vi "Build SMU Waveform.vi"(0 "Measure Load Current":T1, 5 "Record Length":i32, 7 "Source Delay":dbl) -> (4 "SMU Waveform":cluster{dbl[], dbl[]})   [LabVIEW 2020, in "LDO Load Transient.lvlib"]
uses:
  LDO Load Transient.lvlib
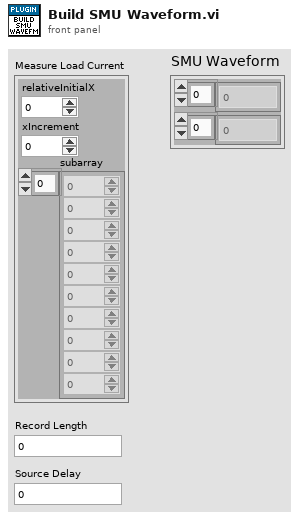
[diagram p1: front panel]
types:
  T1 = cluster{"relativeInitialX":dbl, "xIncrement":dbl, "subarray":dbl[]}
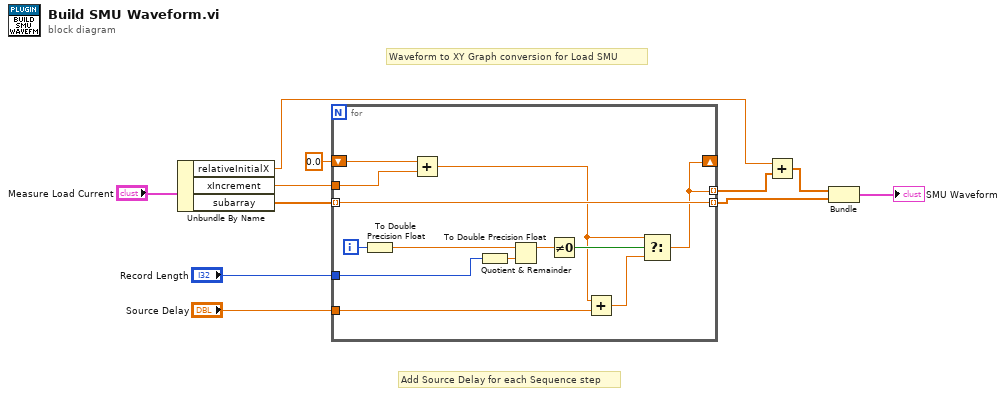
[diagram p0: block diagram]
diagram:
  # "Waveform to XY Graph conversion for Load SMU"
  # "Add Source Delay for each Sequence step"
  n1 = Unbundle By Name("Measure Load Current") -> ("relativeInitialX"=w1:dbl, "xIncrement"=w11:dbl, "subarray"=w10:dbl[])
  n2 = for {
    tunnel: w11 -> [w15]
    tunnel: [w23] -> w5 mode=indexing
    tunnel: [w12] -> w3 mode=indexing
    tunnel: w10 -> [w23] mode=indexing
    tunnel: "Record Length" -> [w21]
    tunnel: "Source Delay" -> [w17]
    shift-right: [w12] -> _
    shift-left: 0.0 -> [w13]
    i -> [w24]
    n3 = To Double Precision Float(number=w24) -> (double precision float=w22:dbl)
    n4 = Add(x=w13, y=w15) -> (x+y=w14:dbl)
    n5 = To Double Precision Float(number=w21) -> (double precision float=w20:dbl)
    n6 = Quotient & Remainder(x=w22, y=w20) -> (x-y*floor(x/y)=w19:dbl)  [unwired: 1 out]
    n7 = Not Equal To 0?(x=w19) -> (x != 0?=w18:bool)
    n8 = Add(x=w14, y=w17) -> (x+y=w16:dbl)
    n9 = Select(t=w14, s=w18, f=w16) -> (s? t:f=w12:dbl)
  }
  n10 = Add(x=w1, y=w3) -> (x+y=w2:dbl[])
  n11 = Bundle(w2, w5) -> (→"SMU Waveform":cluster{dbl[], dbl[]})  [unwired: 1 in]
